vi "Model - Init.vi"(8 "error in (no error)":errorcluster) -> (0 "error out":errorcluster, 3 "View Model":T1)   [LabVIEW 2017]
doc: "Initialize all View Model components"
uses:
  Controls/View Model.ctl
  Configuration/Controls/Config Model.ctl
  Configuration/Controls/Config Data.ctl
  Error Handler/Controls/Error Model.ctl
  Error Handler/Controls/Error Data.ctl
  Error Handler/Controls/Error Type.ctl
  Controls/Shared Model.ctl
  Elevator Controller/Controls/Elevator Model.ctl
  Elevator Controller/Controls/Elevator Location.ctl
  Elevator Controller/Controls/Elevator CMD Data.ctl
  Elevator Controller/Controls/Elevator Commands.ctl
  Elevator Controller/Controls/Elevator Overhead.ctl
  Elevator Controller/Controls/Elevator States.ctl
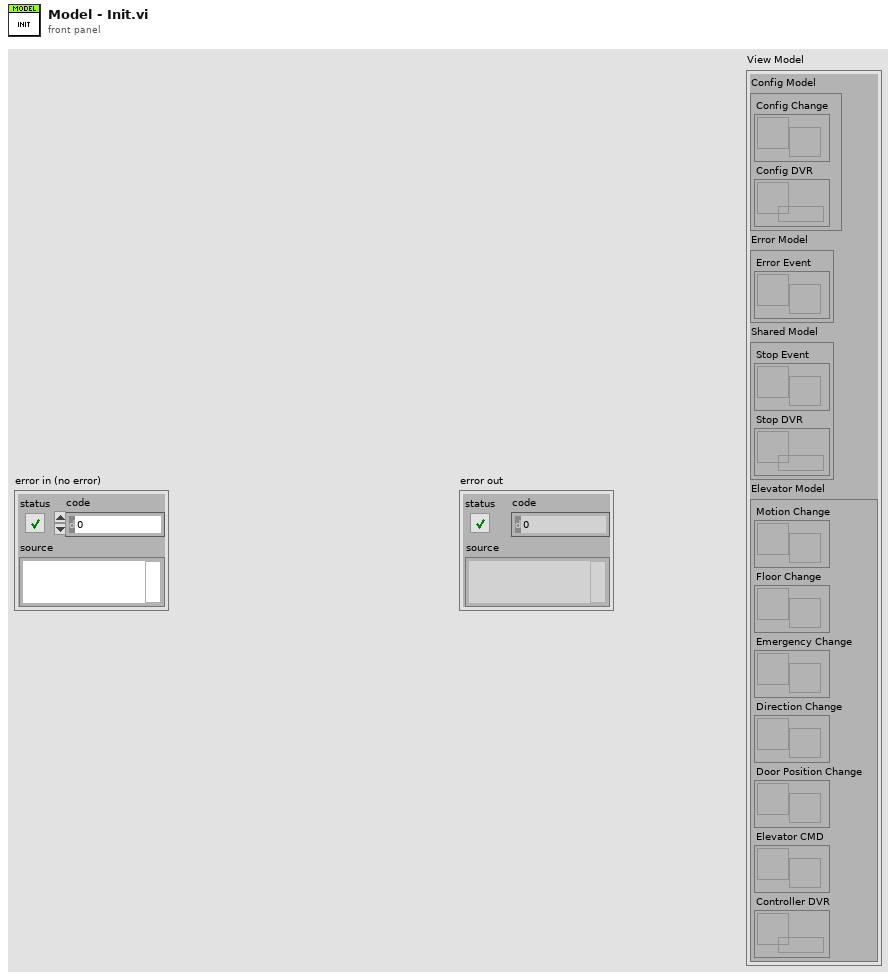
[diagram p1: front panel]
types:
  T1 = typedef "View Model.ctl" = cluster{"Config Model":T2, "Error Model":T3, "Shared Model":T4, "Elevator Model":T5}
  T2 = typedef "Config Model.ctl" = cluster{"Config Change":refnum<user-event>, "Config DVR":refnum<data-value>}
  T3 = typedef "Error Model.ctl" = cluster{"Error Event":refnum<user-event>}
  T4 = typedef "Shared Model.ctl" = cluster{"Stop Event":refnum<user-event>, "Stop DVR":refnum<data-value>}
  T5 = typedef "Elevator Model.ctl" = cluster{"Motion Change":refnum<user-event>, "Floor Change":refnum<user-event>, "Emergency Change":refnum<user-event>, "Direction Change":refnum<user-event>, "Door Position Change":refnum<user-event>, "Elevator CMD":refnum<user-event>, "Controller DVR":refnum<data-value>}
  T6 = typedef "Elevator Location.ctl" = enum16{"1st Floor", "2nd Floor", "3rd Floor", "4th Floor"}
  T7 = typedef "Elevator CMD Data.ctl" = cluster{"Elevator Commands":T8, "Variant":variant}
  T8 = typedef "Elevator Commands.ctl" = enum16{"Go Up", "Go Down", "Go to Floor", "Open Doors", "Close Doors", "Emergency"}
  T9 = typedef "Elevator Overhead.ctl" = cluster{"In Motion?":bool, "Direction":bool, "Door Movement":bool, "Door Position":bool, "Timer":dbl, "Elapsed Time":dbl, "Elevator State":T10, "Elevator Next State":T10}
  T10 = typedef "Elevator States.ctl" = enum16{"Initial", "Wait for 1st Request", "Start and Move", "Analysis", "Continue Travel", "Stop at Floor", "Open and Close Door", "No Request", "Emergency", "Terminate"}
  T11 = typedef "Error Data.ctl" = cluster{"Error Type":T12, "Variant":variant}
  T12 = typedef "Error Type.ctl" = enum16{"Console Error", "Sensor Interface IO Error", "Process Step Error"}
  T13 = typedef "Config Data.ctl" = cluster{"Door Open":dbl, "Door Close":dbl, "Travel Time":dbl, "Inactivity Time":dbl}
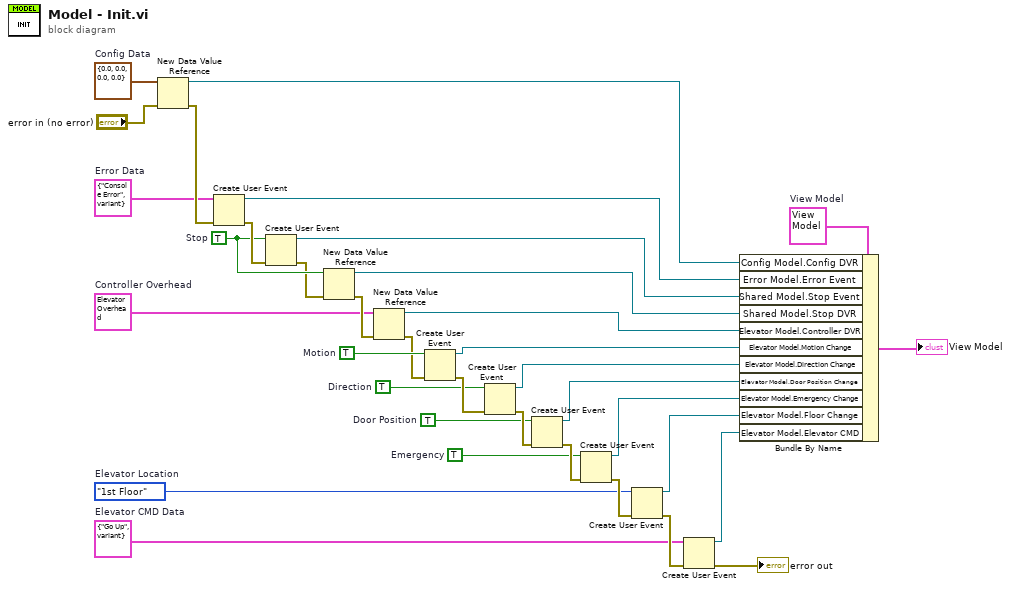
[diagram p0: block diagram]
diagram:
  w2 = Elevator_Location."1st Floor"  # Elevator Location
  w3 = T7 {"Elevator Commands"=enum."Go Up", "Variant"=variant}  # Elevator CMD Data
  w4 = T9 {"In Motion?"=FALSE, "Direction"=FALSE, "Door Movement"=FALSE, "Door Position"=FALSE, "Timer"=0.0, "Elapsed Time"=0.0, "Elevator State"=enum."Initial", "Elevator Next State"=enum."Initial"}  # Controller Overhead
  w5 = T11 {"Error Type"=enum."Console Error", "Variant"=variant}  # Error Data
  w6 = T13 {"Door Open"=0.0, "Door Close"=0.0, "Travel Time"=0.0, "Inactivity Time"=0.0}  # Config Data
  w7 = T1 {"Config Model"={"Config Change"=refnum, "Config DVR"=refnum}, "Error Model"={"Error Event"=refnum}, "Shared Model"={"Stop Event"=refnum, "Stop DVR"=refnum}, "Elevator Model"={"Motion Change"=refnum, "Floor Change"=refnum, "Emergency Change"=refnum, "Direction Change"=refnum, "Door Position Change"=refnum, "Elevator CMD"=refnum, "Controller DVR"=refnum}}  # View Model
  w24 = TRUE  # Emergency
  w26 = TRUE  # Door Position
  w28 = TRUE  # Direction
  w31 = TRUE  # Motion
  w34 = TRUE  # Stop
  n1 = New Data Value Reference(data value=w6, error in="error in (no error)") -> (data value reference=w10:refnum<data-value>, error out=w11:errorcluster)
  n2 = Create User Event(user event datatype=w5, error in=w11) -> (user event=w21:refnum<user-event>, error out=w35:errorcluster)
  n3 = Create User Event(user event datatype=w34, error in=w35) -> (user event=w20:refnum<user-event>, error out=w33:errorcluster)
  n4 = New Data Value Reference(data value=w34, error in=w33) -> (data value reference=w19:refnum<data-value>, error out=w32:errorcluster)
  n5 = New Data Value Reference(data value=w4, error in=w32) -> (data value reference=w18:refnum<data-value>, error out=w30:errorcluster)
  n6 = Create User Event(user event datatype=w31, error in=w30) -> (user event=w17:refnum<user-event>, error out=w29:errorcluster)
  n7 = Create User Event(user event datatype=w28, error in=w29) -> (user event=w16:refnum<user-event>, error out=w27:errorcluster)
  n8 = Create User Event(user event datatype=w26, error in=w27) -> (user event=w15:refnum<user-event>, error out=w25:errorcluster)
  n9 = Create User Event(user event datatype=w24, error in=w25) -> (user event=w14:refnum<user-event>, error out=w23:errorcluster)
  n10 = Create User Event(user event datatype=w2, error in=w23) -> (user event=w13:refnum<user-event>, error out=w22:errorcluster)
  n11 = Create User Event(user event datatype=w3, error in=w22) -> (user event=w12:refnum<user-event>, error out=→"error out":errorcluster)
  n12 = Bundle By Name(cluster=w7, "Config Model.Config DVR"=w10, "Error Model.Error Event"=w21, "Shared Model.Stop Event"=w20, "Shared Model.Stop DVR"=w19, "Elevator Model.Controller DVR"=w18, "Elevator Model.Motion Change"=w17, "Elevator Model.Direction Change"=w16, "Elevator Model.Door Position Change"=w15, "Elevator Model.Emergency Change"=w14, "Elevator Model.Floor Change"=w13, "Elevator Model.Elevator CMD"=w12) -> (→"View Model":T1)
